vi "Post New Tweet - Finite.vi"() -> ()   [LabVIEW 2011]
doc: "This example posts a text only tweet."
uses:
  i3-twitter.lvlib
panel:
  in  "Tweet":string
  in  "Consumer Secret":string
  in  "Consumer Key":string
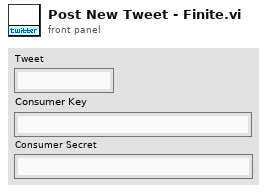
[diagram p1: front panel]
types:
  T1 = typedef "i3-twitter.lvlib/Twitter Handle.ctl" = cluster{"OAuth Credentials":T2, "since ID":string, "max ID":string, "Screen Name":string}
  T2 = typedef "i3-oauth.lvlib/OAuth Credentials.ctl" = cluster{"Consumer Key":string, "Signature Method":T3, "Token":string, "Version":string, "Token Secret":string, "Consumer Secret":string}
  T3 = typedef "i3-oauth.lvlib/Signature Method.ctl" = enum16{"HMAC-MD5", "HMAC-SHA1", "HMAC-SHA224", "HMAC-SHA256", "HMAC-SHA384", "HMAC-SHA512"}
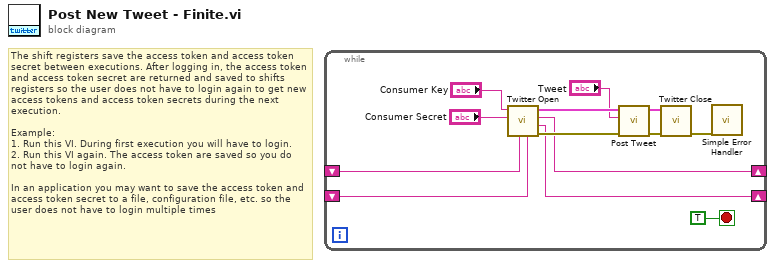
[diagram p0: block diagram]
diagram:
  # "The shift registers save the access token and access token secret between executions. After logging in, the access token and access token secret are returned and saved to shifts registers so the user does not have to login again to get new access tokens and access token secrets during the next execution.\n\nExample:\n1. Run this VI. During first execution you will have to login.\n2. Run this VI again. The access token are saved so you do not have to login again.\n\nIn an application you may want to save the access token and access token secret to a file, configuration file, etc. so the user does not have to login multiple times"
  n1 = while {
    shift-right: [w6] -> _
    shift-left: _ -> [w1]
    shift-right: [w5] -> _
    shift-left: _ -> [w2]
    stop <- TRUE stop-if-true
    n2 = call "Twitter Open.vi"("Access Token Secret (In)"=w2, "Access Token (In)"=w1, "Consumer Secret"="Consumer Secret", "Consumer Key"="Consumer Key") -> ("error out"=w13:errorcluster, "Access Token Secret (Out)"=w5:string, "Access Token (Out)"=w6:string, "Twitter Handle Out"=w11:T1)  [unwired: 4 in]
    n3 = call "Post Tweet.vi"("error in (no error)"=w13, "Tweet"="Tweet", "Twitter Handle In"=w11) -> ("error out"=w12:errorcluster, "Twitter Handle Out"=w10:T1)  [unwired: 7 in]
    n4 = call "Twitter Close.vi"("error in"=w12, "Twitter Handle In"=w10) -> ("error in"=w3:errorcluster)  [unwired: 9 in]
    n5 = call <vilib>:"Simple Error Handler.vi"("error in (no error)"=w3) -> ()  [unwired: 4 in, 5 out]
  }
